vi "ConfigureFPGA.vi"(8 "Status/Errors in":refnum<vi>, 10 "RBF file path in":path) -> (0 "Status/Errors out":refnum<vi>, 2 "RBF file path out":string)   [LabVIEW 2010]
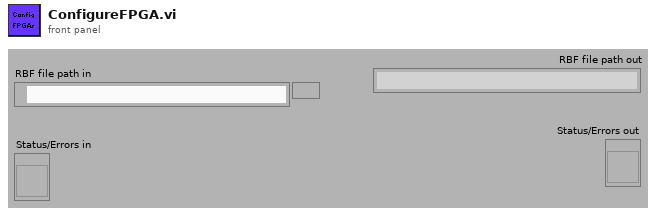
[diagram p1: front panel]
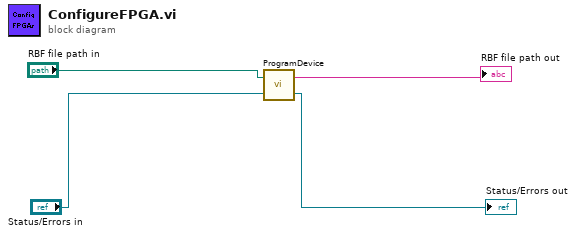
[diagram p0: block diagram]
diagram:
  n1 = call "ProgramDevice.vi"("Status/Errors in"="Status/Errors in", "RBF file path in"="RBF file path in") -> ("Status/Errors out"=→"Status/Errors out":refnum<vi>, "RBF file path out"=→"RBF file path out":string)
